vi "Ping Tree.vi"(8 "error in (no error)":errorcluster, 11 "UI_Actor in":refnum<class "UI_Actor.lvclass">) -> (0 "error out":errorcluster, 3 "UI_Actor out":refnum<class "UI_Actor.lvclass">)   [LabVIEW 2020, in "UI_Actor.lvlib" / "UI_Actor.lvclass"]
uses:
  UI_Actor.lvclass
  D:/Projets/STEP AT/UI Actor/support/Actor Framework.lvlibp/1abvi3w/vi.lib/ActorFramework/Actor/Actor.lvclass
  ctl_Ping payload.ctl
  UI_Actor.lvclass/UI_Actor.ctl
  UI_Actor Messages/Ping core Msg/Ping core Msg.lvclass/Ping core Msg.ctl
  support/Actor Framework.lvlibp/1abvi3w/vi.lib/ActorFramework/Message Enqueuer/Enqueue.vi
  UI_Actor Messages/Ping core Msg/Ping core Msg.lvclass
  support/Actor Framework.lvlibp/1abvi3w/vi.lib/ActorFramework/Actor/Actor.lvclass
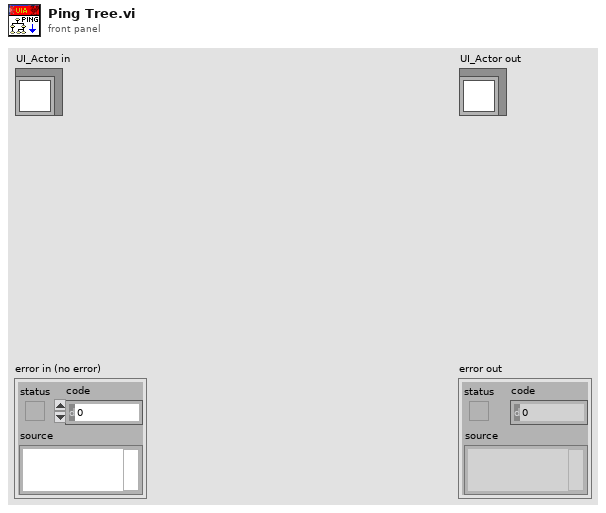
[diagram p1: front panel]
types:
  T1 = typedef "UI_Actor.lvlib/UI_Actor.lvclass/ctl_Ping payload.ctl" = cluster{"Responsible":string, "Time":timestamp}
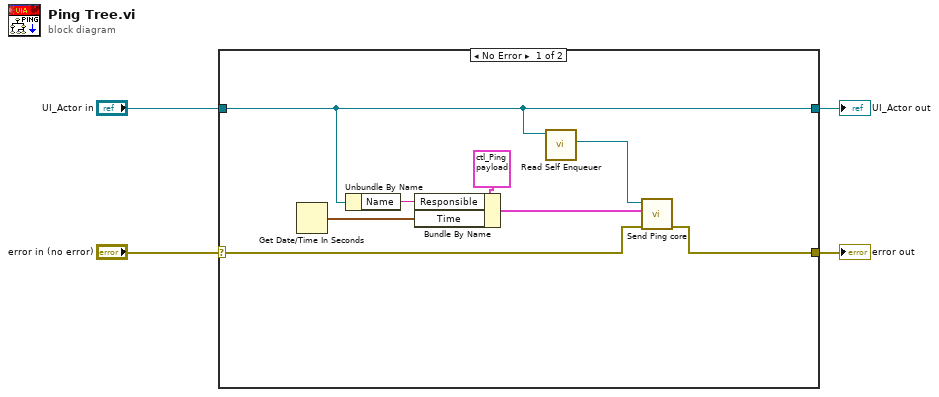
[diagram p0: block diagram]
diagram:
  n1 = case shown="No Error" "error in (no error)" {
    selector: "error in (no error)" -> [w6 w14]
    tunnel: [w5 w14] -> w3
    tunnel: [w7 w13] -> w1
    tunnel: "UI_Actor in" -> [w7 w13]
    frame No Error {
      n2 = Get Date/Time In Seconds() -> (seconds since 1Jan1904=w8:timestamp)
      n3 = Unbundle By Name(w7) -> ("Name"=w9:string)
      n4 = Bundle By Name(cluster=T1 {"Responsible"="", "Time"=timestamp(0 s since 1904-01-01)} ("Ping payload"), "Responsible"=w9, "Time"=w8) -> (w11:T1)
      n5 = call "Read Self Enqueuer.vi"("Actor"=w7) -> ("Self Enqueuer"=w10:refnum<class "Message Enqueuer.lvclass">)  [unwired: 10 in]
      n6 = call "Send Ping core.vi"("error in (no error)"=w6, "Emission"=w11, "Message Enqueuer"=w10) -> ("error out"=w5:errorcluster)  [unwired: 7 in, 1 out]
    }
    frame Error {
    }
  }
  "error out" <- w3
  "UI_Actor out" <- w1
